vi "Real-Time OS Check.vi"(8 "error in":errorcluster, 11 "System Session in":refnum<k21>) -> (0 "error out":errorcluster, 3 "System Session out":refnum<k21>)   [LabVIEW 2016, in "SMI.lvlib" / "SysCfg Device.lvclass"]
uses:
  SysCfg Device.lvclass
  <resource>/objmgr/nisysapi.rc
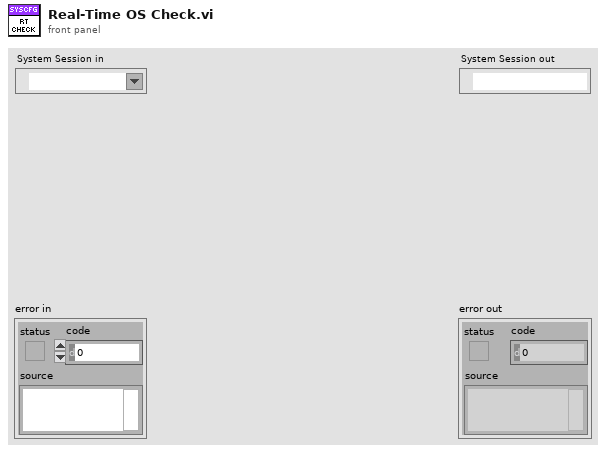
[diagram p1: front panel]
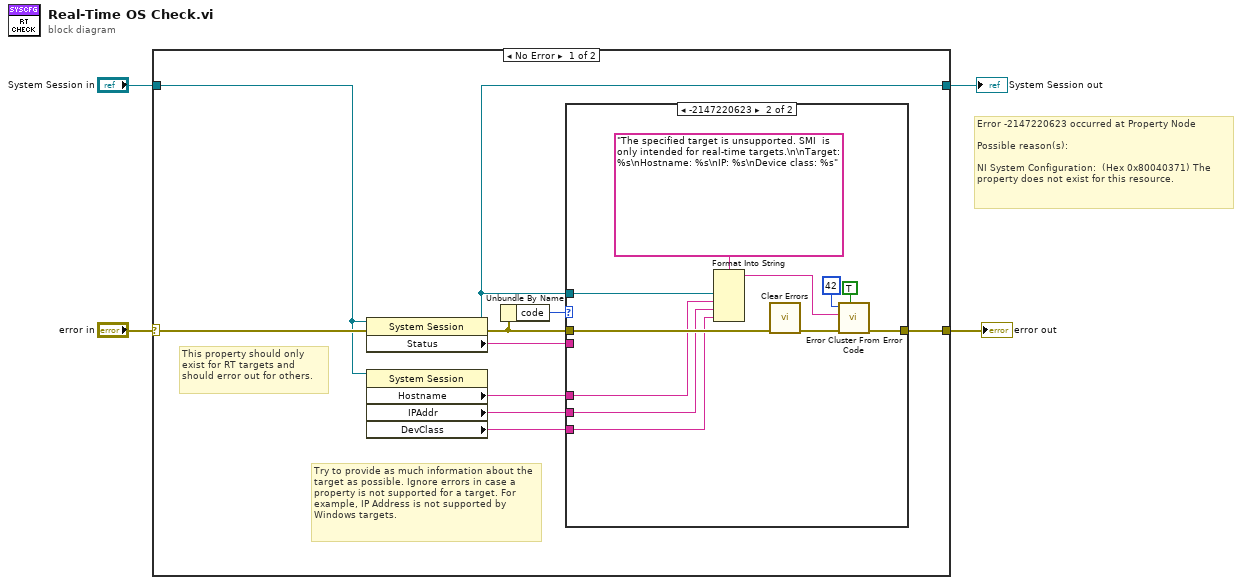
[diagram p0: block diagram]
diagram:
  # "Error -2147220623 occurred at Property Node\n\nPossible reason(s):\n\nNI System Configuration:  (Hex 0x80040371) The property does not exist for this resource."
  n1 = case shown="No Error" "error in" {
    selector: "error in" -> [w14 w28]
    tunnel: [w11 w28] -> w2
    tunnel: "System Session in" -> [w8 w27]
    tunnel: [w9 w27] -> w4
    frame No Error {
      # "Try to provide as much information about the target as possible. Ignore errors in case a property is not supported for a target. For example, IP Address is not supported by Windows targets."
      # "This property should only exist for RT targets and should error out for others."
      n2 = property class="System Session"(reference=w8, error in=w14) -> (reference out=w9:refnum<k21>, error out=w12:errorcluster, "Status"=w10:string)
      n3 = property class="System Session"(reference=w8) -> ("Hostname"=w7:string, "IPAddr"=w6:string, "DevClass"=w5:string)  [unwired: 1 in, 2 out]
      n4 = Unbundle By Name(w12) -> ("code"=w13:i32)
      n5 = case shown="-2147220623" w13 {
        tunnel: w12 -> [w15 w26]
        tunnel: [w15 w24] -> w11
        tunnel: w10 -> [_ _]
        tunnel: w9 -> [_ w20]
        tunnel: w7 -> [_ w19]
        tunnel: w6 -> [_ w18]
        tunnel: w5 -> [_ w17]
        frame Default {
        }
        frame -2147220623 {
          n6 = Format Into String(format string="The specified target is unsupported. SMI  is only intended for real-time targets.\n\nTarget: %s\nHostname: %s\nIP: %s\nDevice class: %s" ("error message (\"\")"), w20, w19, w18, w17) -> (resulting string=w22:string)  [unwired: 2 in, 1 out]
          n7 = call <vilib>:"Clear Errors.vi"("error in (no error)"=w26) -> ("error out"=w25:errorcluster)  [unwired: 5 in, 1 out]
          n8 = call <vilib>:"Error Cluster From Error Code.vi"("show call chain? (False)"=TRUE, "error in (no error)"=w25, "error message (\"\")"=w22, "error code (0)"=42) -> ("error out"=w24:errorcluster)  [unwired: 5 in]
        }
      }
    }
    frame Error {
    }
  }
  "error out" <- w2
  "System Session out" <- w4
